vi "BlockShot.vi"(0 "object in":refnum<class "DefendGoalTactic.lvclass">, 2 "Robot":refnum<class "Robot.lvclass">, 4 "Game":refnum<class "Game.lvclass">, 5 "error in (no error)":errorcluster, 7 "first call?":bool) -> (14 "object out":refnum<class "DefendGoalTactic.lvclass">, 16 "Robot out":refnum<class "Robot.lvclass">, 19 "error out":errorcluster)   [LabVIEW 2024, in "DefendGoalTactic.lvclass"]
uses:
  DefendGoalTactic.lvclass
  Robot_class/Robot.lvclass
  C:/Users/as119/OneDrive/Documentos/roboIME/SSL_AI/Object_class/Object.lvclass
  Game_class/Game.lvclass
  Game_class/Game.lvclass/Game.ctl
  Object_class/Object.lvclass/Object.ctl
  Parameters_class/Parameters.lvclass/Parameters.ctl
  Ball_class/Ball.lvclass/Ball.ctl
  Field_class/Field.lvclass/Field.ctl
  Robot_class/Robot.lvclass/Robot.ctl
  <vilib>/Analysis/_algsub.llb/Real Vector Norm.vi
  Field_class/Read ourGoalPosition.vi
  Parameters_class/Read KickForce.vi
  Parameters_class/Read ChipKick Force 1.vi
  Object_class/Read position(x,y).vi
  Ball_class/Read v_x.vi
  Ball_class/Read v_y.vi
  Ball_class/Read velocityNorm.vi
  Robot_class/Write dest_vel.vi
  Robot_class/Write dest_x.vi
  Robot_class/Write dest_y.vi
  Robot_class/Write dest_orientation.vi
  Robot_class/Write kick_x.vi
  Robot_class/Write kick_z.vi
  Game_class/Read FieldRef.vi
  Game_class/Read BallRef.vi
  Game_class/Read Parameters.lvclass.vi
  Game_class/Read NewParameters.vi
  Ball_class/Ball.lvclass
  Field_class/Field.lvclass
  Parameters_class/Parameters.lvclass
  Utilities_class/Utilities.lvclass
  <vilib>/Analysis/NI_AALPro.lvlib
  <vilib>/Analysis/NI_AALBLAS.lvlib
  <vilib>/Analysis/coordinate.llb/2D Cartesian Coordinate Rotation (Scalar).vi
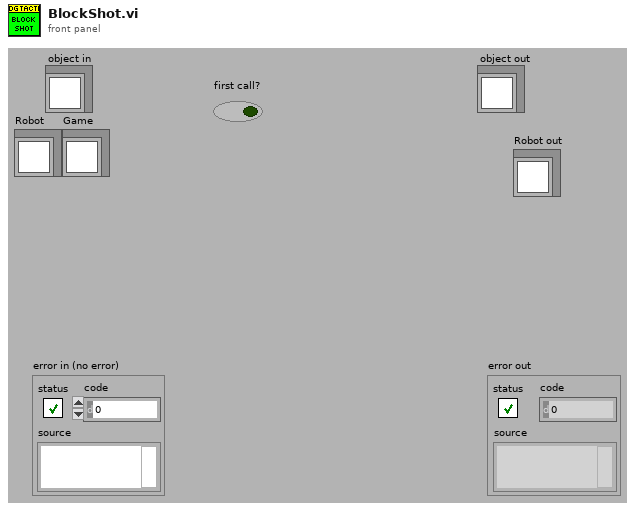
[diagram p1: front panel]
types:
  T1 = typedef "NewParameters.ctl" = cluster{"PenaltyDistance":dbl, "DistanceAttackerToBackBall":dbl, "Division":enum16{"Div B", "Div A"}, "DistanceToAvoidyEnemyRobot":dbl, "BallPlacementDistance":dbl, "DisatanceBehindBallToStealBall":dbl, "MaxDistanceToPositionKickoff":dbl, "BlockEnemyTarget":bool, "MaxStopVAng":dbl, "DistanceMarkerToEnemy":dbl, "IgnoreDribblerContact":bool, "DistanceToBeginEnemyPosession":dbl, "GoToBallWhenEnemyNotMoving":bool, "EnemyDistanceToReduceVelocity":dbl, "TurnOnEnemyDistanceToReduceVelocity":bool, "EnemyDistanceToShootOutBall":dbl, "DefenseKickBall":bool, "MoreKickToGoal? (0-0.3)":dbl, "ChipKickInEnemyField":bool, "ShootOutRobotId":dbl, "FieldLenghtDenominatorInShootOut":dbl, "AdjustPositionInBallPlacement":bool, "PowerGodPass":dbl, "VelocityAbortEnemyPos":dbl, "MaxDistToBeginPass":dbl, "MinDistToBeginPass":dbl, "VelocityInDirects":dbl, "BadDribblerIDs":i32[], "NewKickToDistanceAroundBall":dbl, "PowerAvoidColisionMarker":dbl, "DistanceToAvoidColisionMarker":dbl, "AvoidBallKick":dbl, "DistanceTryKick":dbl, "SuicideKickDIstance":dbl, "AdjustFirstKickDistance":dbl, "AvoidAimLessKick":dbl, "DistanceToAvoidyEnemyShootRobot ":dbl, "NumberOfMarkers":dbl, "PotField":bool, "PIDLateral":bool, "MinDistanceFirstKickX":dbl, "MinDistanceFirstKickY":dbl, "FractionOfDistToTouchGround\nAfterChipKick":dbl, "FractionOfKickxWhen\nComposedWithKickz":dbl, "Style":T2, "MoveInTurnState":bool, "DistFromEnemyToConsider\nMoveInTurnState":dbl, "CascadePID":bool, "TurnAroundParameters":cluster{"Radius":dbl, "Multiplier":dbl, "ChordAngle":dbl}, "SafeDriveVel":dbl, "DistanceToGoToBackBall":dbl, "minDistanceToNotFinish\nEnemyPossession":dbl, "OneTouchShot":cluster{"angleFactor":dbl, "maxAngle":dbl, "Attack":bool, "Defense":bool}, "OpenAngleToGoal":cluster{"minAngle":dbl, "maxAngle":dbl, "minEvaluation":dbl}, "ShotInterception":cluster{"shotSpeed":dbl, "minEnemySpeed":dbl, "maxEnemySpeed":dbl, "minEvaluation":dbl}, "AllyTeamArray":T3[], "maxDefendersNumber":i32, "Zone":cluster{"GuardPositionArray":dbl[][], "ZoneMidField":dbl[], "CenterForwardWidth":dbl}, "MinEvaluationToShoot":dbl, "PassInterception":cluster{"maxPassSpeed":dbl, "minPassSpeed":dbl, "minEnemySpeed":dbl, "chipPassDistance":dbl, "chipPassEvaluation":dbl, "minEvaluation":dbl, "maxEnemySpeed":dbl}, "PassDistance":cluster{"maxDistance":dbl, "minDistance":dbl}, "receiverSpeed":dbl, "maxBallSpeed":dbl, "slackTime":dbl, "Turning radius":dbl, "Turning v_ang":dbl, "AlignError":cluster{"Distance":dbl, "Orientation":dbl, "V_norm(m/s)":dbl, "V_ang (rad/s)":dbl}, "RobotRadius":dbl, "KickerDistance":dbl, "keeper angle  to cover goalpost":dbl, "a_slide":dbl, "a_roll":dbl, "k_switch":dbl}
  T2 = typedef "Style.ctl" = enum16{"Insanity", "Offensive", "Defensive"}
  T3 = typedef "AllyTeam.ctl" = enum16{"Keeper", "Defender", "Attacker"}
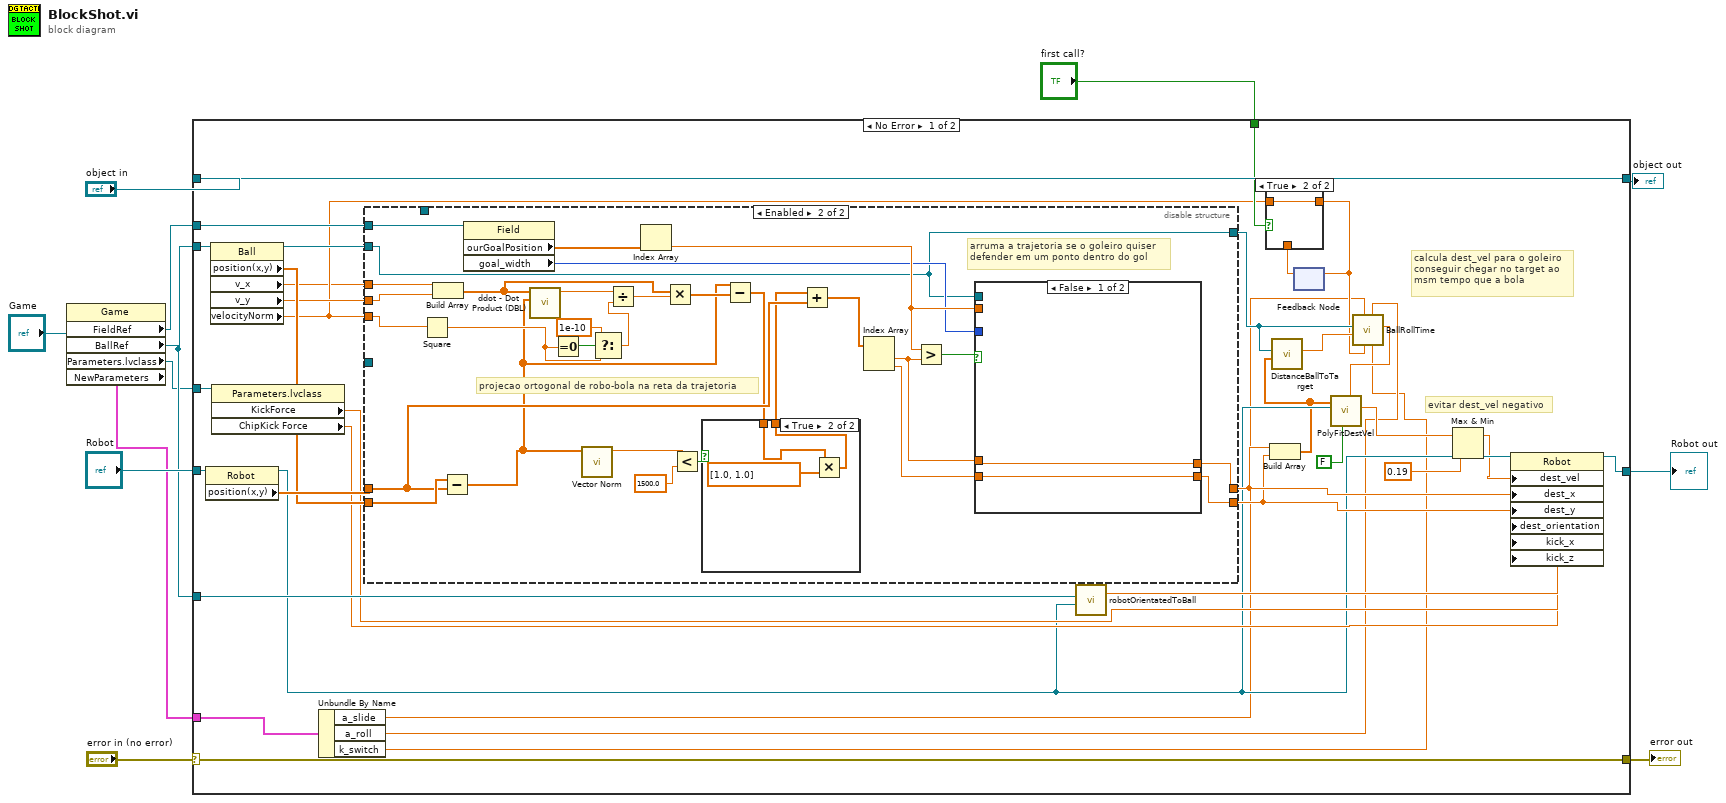
[diagram p0: block diagram]
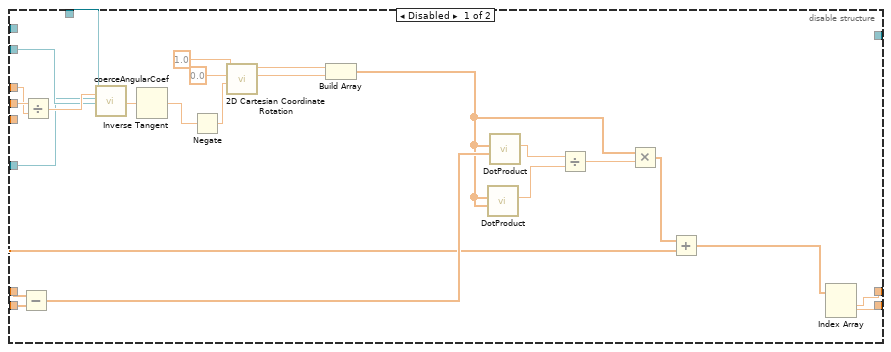
[diagram p3: hidden frame]
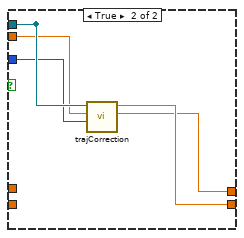
[diagram p5: hidden frame]
diagram:
  n1 = property class="Game"(reference="Game") -> ("FieldRef"=w4:refnum<class "Field.lvclass">, "BallRef"=w5:refnum<class "Ball.lvclass">, "Parameters.lvclass"=w3:refnum<class "Parameters.lvclass">, "NewParameters"=w1:T1)  [unwired: 1 in, 2 out]
  n2 = case shown="No Error" "error in (no error)" {
    selector: "error in (no error)" -> [w47 w117]
    tunnel: [w47 w117] -> w11
    tunnel: [w42 w116] -> w9
    tunnel: "object in" -> [w42 w116]
    tunnel: "Robot" -> [w46 w115]
    tunnel: w5 -> [w45 _]
    tunnel: [w44 w115] -> w6
    tunnel: w5 -> [w39 _]
    tunnel: w4 -> [w38 _]
    tunnel: w3 -> [w36 _]
    tunnel: "first call?" -> [w24 _]
    tunnel: w1 -> [w16 _]
    frame No Error {
      # "calcula dest_vel para o goleiro\nconseguir chegar no target ao\nmsm tempo que a bola"
      # "evitar dest_vel negativo"
      n3 = property class="Robot"(reference=w46) -> (reference out=w29:refnum<class "Robot.lvclass">, "position(x,y)"=w41:dbl[])  [unwired: 1 in, 1 out]
      n4 = property class="Ball"(reference=w45) -> (reference out=w37:refnum<class "Ball.lvclass">, "position(x,y)"=w40:dbl[], "v_x"=w18:dbl, "v_y"=w33:dbl, "velocityNorm"=w19:dbl)  [unwired: 1 in, 1 out]
      n5 = property class="Parameters.lvclass"(reference=w36) -> ("KickForce"=w35:dbl, "ChipKick Force"=w34:dbl)  [unwired: 1 in, 2 out]
      n6 = Unbundle By Name(w16) -> ("a_slide"=w15:dbl, "a_roll"=w14:dbl, "k_switch"=w13:dbl)
      n7 = disable-structure shown="Enabled" {
        disable-tunnel: _ -> [w72 _]
        disable-tunnel: w37 -> [w71 w80]
        disable-tunnel: _ -> [w70 _]
        disable-tunnel: w33 -> [w64 w102]
        disable-tunnel: w18 -> [w63 w103]
        disable-tunnel: w41 -> [w62 w94]
        disable-tunnel: w40 -> [w56 w95]
        disable-tunnel: [w53 w87] -> w31
        disable-tunnel: [w52 w86] -> w30
        disable-tunnel: w19 -> [_ w101]
        disable-tunnel: w38 -> [_ w90]
        disable-tunnel: [_ w80] -> w28
        frame Disabled {
          n8 = Subtract(x=w62, y=w56) -> (x-y=w61:dbl[])
          n9 = Divide(x=w64, y=w63) -> (x/y=w73:dbl)
          n10 = call "coerceAngularCoef.vi"("object in"=w72, "Coef ang"=w73, "Field"=w70, "Ball"=w71) -> ("coerced(x)"=w67:dbl)  [unwired: 13 in, 2 out]
          n11 = Inverse Tangent(1:w67) -> (0:w51:dbl)
          n12 = Negate(x=w51) -> (-x=w50:dbl)
          n13 = call-poly <vilib>:"2D Cartesian Coordinate Rotation.vi"("theta"=w50, "y"=0.0, "x"=1.0) -> ("y out"=w65:dbl, "x out"=w66:dbl)  [unwired: 6 in, 1 out]
          n14 = Build Array(w66, w65) -> (w57:dbl[])
          n15 = call "DotProduct.vi"("Point2"=w57, "Point1"=w57) -> ("dot product"=w59:dbl)  [unwired: 7 in, 2 out]
          n16 = call "DotProduct.vi"("Point2"=w61, "Point1"=w57) -> ("dot product"=w60:dbl)  [unwired: 7 in, 2 out]
          n17 = Divide(x=w60, y=w59) -> (x/y=w58:dbl)
          n18 = Multiply(x=w57, y=w58) -> (x*y=w55:dbl[])
          n19 = Add(x=w55, y=w56) -> (x+y=w54:dbl[])
          n20 = Index Array(array=w54) -> (element #1=w53:dbl, element #2=w52:dbl)  [unwired: 2 in]
        }
        frame Enabled {
          # "arruma a trajetoria se o goleiro quiser \ndefender em um ponto dentro do gol"
          # "projecao ortogonal de robo-bola na reta da trajetoria"
          n21 = Square(x=w101) -> (x^2=w83:dbl)
          n22 = Build Array(w103, w102) -> (w98:dbl[])
          n23 = Subtract(x=w95, y=w94) -> (x-y=w79:dbl[])
          n24 = property class="Field"(reference=w90) -> ("ourGoalPosition"=w89:dbl[], "goal_width"=w85:i32)  [unwired: 1 in, 2 out]
          n25 = call <vilib>:"ddot - Dot Product (DBL).vi"("y"=w79, "x"=w98) -> ("ddot"=w100:dbl)  [unwired: 8 in, 1 out]
          n26 = Equal To 0?(x=w83) -> (x = 0?=w84:bool)
          n27 = call-poly <vilib>:"Vector Norm.vi"("Input Vector"=w79) -> ("norm"=w78:dbl)  [unwired: 9 in, 1 out]
          n28 = Select(t=1e-10, s=w84, f=w83) -> (s? t:f=w82:dbl)
          n29 = Divide(x=w100, y=w82) -> (x/y=w99:dbl)
          n30 = Index Array(array=w89) -> (element=w88:dbl)  [unwired: 1 in]
          n31 = Multiply(x=w98, y=w99) -> (x*y=w97:dbl[])
          n32 = Less?(x=w78, y=1500.0) -> (x < y?=w76:bool)
          n33 = Subtract(x=w79, y=w97) -> (x-y=w74:dbl[])
          n34 = case shown="True" w76 {
            tunnel: [w104 w105] -> w75
            tunnel: w74 -> [w104 w107]
            frame False {
            }
            frame True {
              n35 = Multiply(x=w107, y=dbl[] [1.0, 1.0]) -> (x*y=w105:dbl[])
            }
          }
          n36 = Add(x=w75, y=w94) -> (x+y=w96:dbl[])
          n37 = Index Array(array=w96) -> (element #1=w91:dbl, element #2=w92:dbl)  [unwired: 2 in]
          n38 = Greater?(x=w88, y=w91) -> (0:w93:bool)
          n39 = case shown="False" w93 {
            tunnel: w92 -> [w108 _]
            tunnel: w91 -> [w109 _]
            tunnel: w88 -> [_ w113]
            tunnel: [_ w114] -> _
            tunnel: w80 -> [_ w114]
            tunnel: [w109 w111] -> w87
            tunnel: [w108 w112] -> w86
            tunnel: w85 -> [_ w110]
            frame False {
            }
            frame True {
              n40 = call "trajCorrection.vi"("goal Width"=w110, "goal X"=w113, "BallRef"=w114) -> ("x"=w111:dbl, "y"=w112:dbl)  [unwired: 6 in]
            }
          }
        }
      }
      n41 = call "robotOrientatedToBall.vi"("Robot"=w29, "BallRef"=w39) -> ("Orientation"=w43:dbl)  [unwired: 7 in, 2 out]
      n42 = Build Array(w31, w30) -> (w27:dbl[])
      n43 = call "DistanceBallToTarget.vi"("Target"=w27, "Ball"=w28) -> ("Distance Ball To Target"=w26:dbl)  [unwired: 7 in, 2 out]
      n44 = feedback #1() -> (w23:dbl)  [unwired: 1 in]
      n45 = case shown="True" w24 {
        tunnel: w19 -> [_ w49]
        tunnel: [w48 w49] -> w22
        tunnel: w23 -> [w48 _]
        frame False {
        }
        frame True {
        }
      }
      n46 = feedback-in #1(w22) -> ()
      n47 = call "BallRollTime.vi"("k_switch"=w13, "acc_roll"=w14, "v_ini"=w22, "acc_slide"=w15, "distance"=w26, "Ball"=w28) -> ("time"=w25:dbl)  [unwired: 3 in, 2 out]
      n48 = call "PolyFitDestVel.vi"("TargetTime"=w25, "use model?"=FALSE, "TargetPos"=w27, "Robot"=w29) -> ("vf"=w20:dbl)  [unwired: 5 in, 2 out]
      n49 = Max & Min(x=w20, y=0.19) -> (max(x,y)=w17:dbl)  [unwired: 1 out]
      n50 = property class="Robot"(reference=w29, "dest_vel"=w17, "dest_x"=w31, "dest_y"=w30, "dest_orientation"=w43, "kick_x"=w35, "kick_z"=w34) -> (reference out=w44:refnum<class "Robot.lvclass">)  [unwired: 1 in, 1 out]
    }
    frame Error {
    }
  }
  "error out" <- w11
  "object out" <- w9
  "Robot out" <- w6
